vi "Actor Core.vi"(8 "error in":errorcluster, 11 "Elevator Controller Actor in":refnum<class "Sim User Console Actor.lvclass">) -> (0 "error out":errorcluster, 3 "Actor out":refnum<class "Actor.lvclass">)   [LabVIEW 2022 SP3, in "Sim User Console Actor.lvlib" / "Sim User Console Actor.lvclass"]
doc: "(<B>Filename</B>: Actor Framework.lvlib:Actor.lvclass:Actor Core.vi)\n\nReceives messages to the actor, reacts to them, and initiates any error handling that may shut the actor down.\n\nDescendant classes may override this VI to append parallel tasks for the actor to complete while it handles messages. Overrides use the Call Parent Class Method node."
uses:
  Sim User Console Actor.lvclass
  <vilib>/ActorFramework/Stop Msg/Stop Msg.lvclass
  <vilib>/ActorFramework/Actor/Actor.lvclass
  User Console Actor/User Console Actor/User Console Actor.lvclass
  C:/Workspace/CLA/Elevator AF_2022_2nd/User Console Actor/User Console Actor/User Console Actor.lvclass
  C:/Program Files/National Instruments/LabVIEW 2022/vi.lib/ActorFramework/Actor/Actor.lvclass
  C:/Workspace/CLA/Elevator AF_2022_2nd/Sim User Console Actor/Elevator Controller Actor/Sim User Console Actor.lvclass
  Sim User Console Actor Messages/Read Elevator Call Msg/Read Elevator Call Msg.lvclass
  Elevator Call.ctl
  Floor Selection.ctl
  Door Buttons.ctl
panel:
  in  "Emergency":bool
  in  "Door Buttons":T1
  in  "Floor Selection":T2
  in  "Elevator Call":T3
  # "[Covers: UI1]\n[Covers: UI2]\n[Covers: UI2A] \n[Covers: UI2A1] \n[Covers: UI2A2] \n[Covers: UI2B] \n[Covers: UI2B1] \n[Covers: UI2B2] \n[Covers: UI2C] \n[Covers: UI2C1] \n[Covers: UI2C2] \n[Covers: UI2C3] \n[Covers: UI2D] \n[Covers: UI2D1]"
  # "Fourth Floor"
  # "Third Floor"
  # "Second Floor"
  # "First Floor"
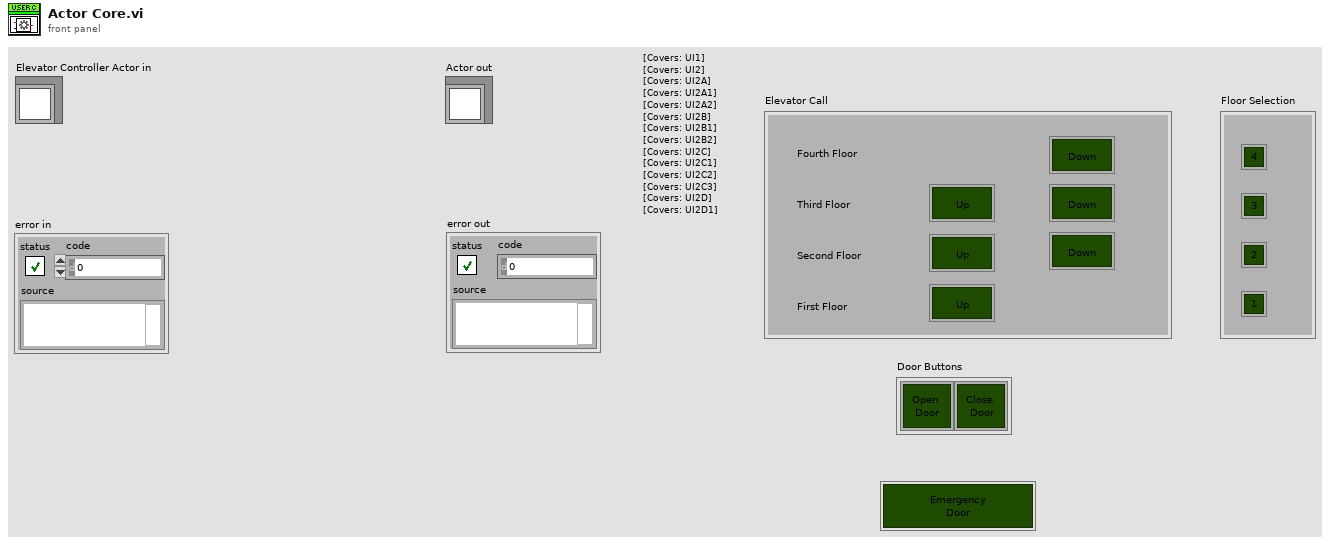
[diagram p1: front panel]
types:
  T1 = typedef "Sim User Console Actor.lvlib/Sim User Console Actor.lvclass/Door Buttons.ctl" = cluster{"Open Door":bool, "Close Door":bool}
  T2 = typedef "Sim User Console Actor.lvlib/Sim User Console Actor.lvclass/Floor Selection.ctl" = cluster{"Floor4":bool, "Floor 3":bool, "Floor2":bool, "Floor1":bool}
  T3 = typedef "Sim User Console Actor.lvlib/Sim User Console Actor.lvclass/Elevator Call.ctl" = cluster{"Up":bool, "Up 2":bool, "Up 3":bool, "Down":bool, "Down 2":bool, "Down 3":bool}
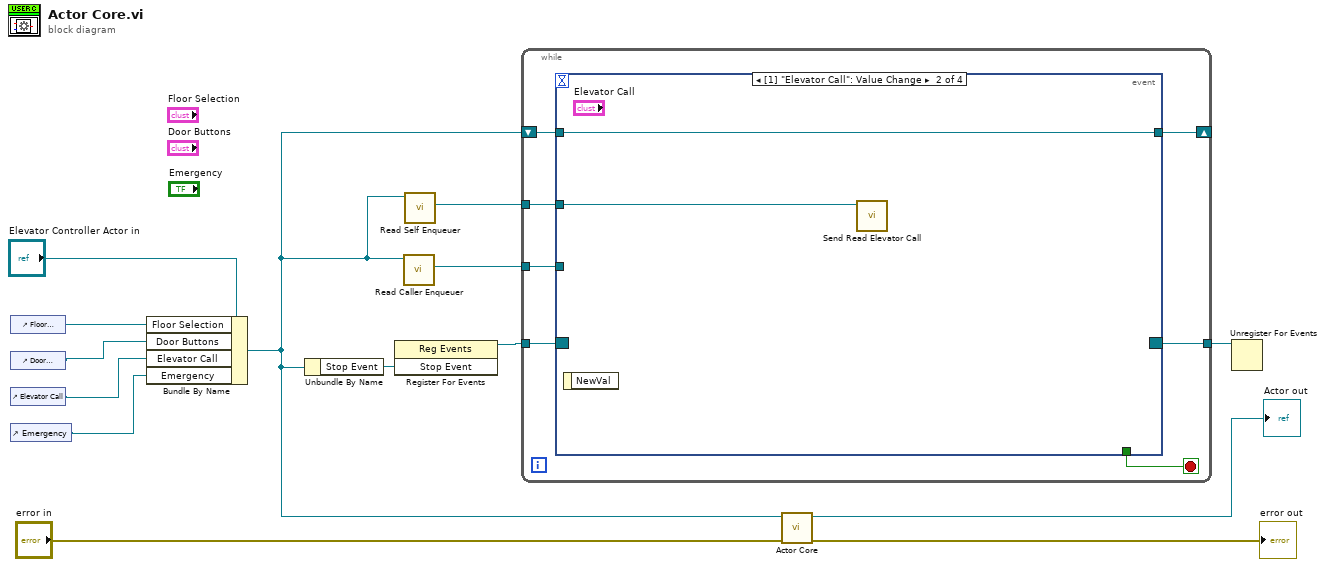
[diagram p0: block diagram]
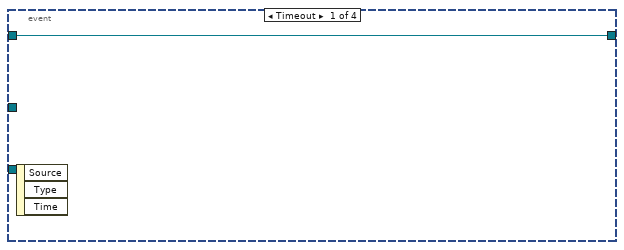
[diagram p2: hidden frame]
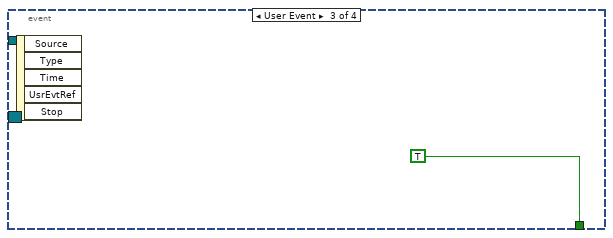
[diagram p3: hidden frame]
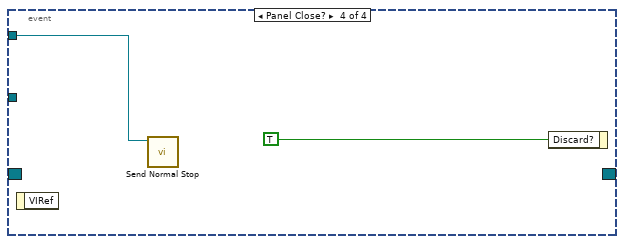
[diagram p4: hidden frame]
diagram:
  n1 = control-ref of="Floor Selection"() -> (w6:refnum<vi>)
  n2 = control-ref of="Door Buttons"() -> (w5:refnum<vi>)
  n3 = control-ref of="Elevator Call"() -> (w4:refnum<vi>)
  n4 = control-ref of="Emergency"() -> (w3:refnum<vi>)
  n5 = Bundle By Name(cluster="Elevator Controller Actor in", "Floor Selection"=w6, "Door Buttons"=w5, "Elevator Call"=w4, "Emergency"=w3) -> (w2:refnum<class "Sim User Console Actor.lvclass">)
  n6 = Unbundle By Name(w2) -> ("Stop Event"=w11:refnum<user-event>)
  n7 = register-events(w11) -> (reference out=w10:refnum<event-registration>)  [unwired: 2 in, 1 out]
  n8 = call <vilib>:"Read Caller Enqueuer.vi"("Actor"=w2) -> ("Caller Enqueuer"=w1:refnum<class "Message Enqueuer.lvclass">)  [unwired: 10 in]
  n9 = call <vilib>:"Read Self Enqueuer.vi"("Actor"=w2) -> ("Self Enqueuer"=w8:refnum<class "Message Enqueuer.lvclass">)  [unwired: 10 in]
  n10 = while {
    tunnel: w10 -> [w20]
    tunnel: [w19] -> w9
    tunnel: w8 -> [w18]
    shift-right: [w16] -> _
    shift-left: w2 -> [w17]
    tunnel: w1 -> [w15]
    stop <- w21 stop-if-true
    n11 = event shown="[1] \"Elevator Call\": Value Change" {
      selector: w20 -> [_ _ _ _]
      dyn-events: [_ _ _ _] -> w19
      timeout: _ -> [_ _ _ _]
      tunnel: [_ _ TRUE _] -> w21
      tunnel: w18 -> [_ w23 _ w26]
      tunnel: w17 -> [w22 w24 _ _]
      tunnel: [w22 w24 _ _] -> w16
      tunnel: w15 -> [_ _ _ _]
      event Timeout {
        n12 = event-data() -> ()  [unwired: 1 in, 3 out]
      }
      event Value Change {
        n13 = event-data() -> ()  [unwired: 1 in, 1 out]
        n14 = call "Send Read Elevator Call.vi"("Message Enqueuer"=w23) -> ()  [unwired: 9 in, 2 out]
      }
      event User Event {
        n15 = event-data() -> ()  [unwired: 1 in, 5 out]
      }
      event Panel Close? {
        n16 = event-data() -> ()  [unwired: 1 in, 1 out]
        n17 = call <vilib>:"Send Normal Stop.vi"("Message Enqueuer"=w26) -> ()  [unwired: 10 in, 1 out]
        n18 = event-data("Discard?"=TRUE) -> ()  [unwired: 1 in, 1 out]
      }
    }
  }
  n19 = call-parent "Actor Core.vi"("error in"="error in", "Actor in"=w2) -> ("error out"=→"error out":errorcluster, "Actor out"=→"Actor out":refnum<class "Actor.lvclass">)  [unwired: 8 in]
  n20 = Unregister For Events(event registration refnum=w9) -> ()  [unwired: 1 in, 1 out]
